vi "624Prepare Joystick Data for Displays.vi"(8 "index Z":i32, 9 "index  y":i32, 10 "index x":i32, 11 "Joystick Values":T1) -> (1 "Buttons":T2, 2 "Z Axis":dbl, 3 "Cartesian Data":cluster{"X axis":dbl, "X axis":dbl}[](array[cluster]))   [LabVIEW 2014]
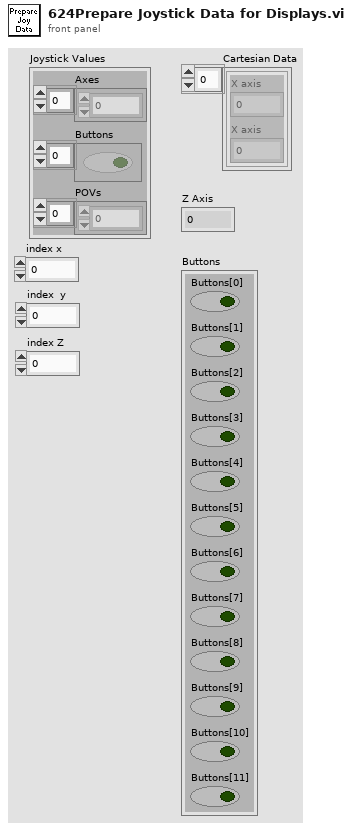
[diagram p1: front panel]
types:
  T1 = cluster{"Axes":dbl[], "Buttons":bool[], "POVs":i16[]}
  T2 = cluster{"Buttons[0]":bool, "Buttons[1]":bool, "Buttons[2]":bool, "Buttons[3]":bool, "Buttons[4]":bool, "Buttons[5]":bool, "Buttons[6]":bool, "Buttons[7]":bool, "Buttons[8]":bool, "Buttons[9]":bool, "Buttons[10]":bool, "Buttons[11]":bool}
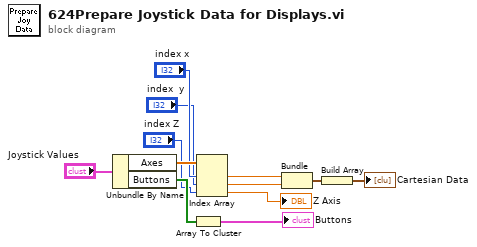
[diagram p0: block diagram]
diagram:
  n1 = Unbundle By Name("Joystick Values") -> ("Axes"=w5:dbl[], "Buttons"=w11:bool[])
  n2 = Array To Cluster(array=w11) -> (cluster=→"Buttons":T2)
  n3 = Index Array(array=w5, index #1="index x", index #2="index  y", index #3="index Z") -> (element #1=w8:dbl, element #2=w9:dbl, element #3=→"Z Axis":dbl)
  n4 = Bundle("X axis"=w8, "X axis"=w9) -> (w7:cluster{"X axis":dbl, "X axis":dbl})  [unwired: 1 in]
  n5 = Build Array(w7) -> (→"Cartesian Data":cluster{"X axis":dbl, "X axis":dbl}[])
